vi "Word - Append Table Tests.vi"(8 "error in (no error)":errorcluster) -> (0 "error out":errorcluster)   [LabVIEW 2017]
uses:
  src/LabVIEW NPOI/MS-Word/MS-Word.lvclass
  C:/Users/Neo/Desktop/Dev_Tools_BR/LabVIEW_NPOI/src/LabVIEW NPOI/Document/Document.lvclass
  src/LabVIEW NPOI/Document/Append Table (string).vi
  src/LabVIEW NPOI/Document/Append Table (double).vi
  <vilib>/addons/_JKI Toolkits/Caraya/classes/Assert/Assert Not Error.vi
  src/LabVIEW NPOI/Document/Document.lvclass
  <vilib>/addons/_JKI Toolkits/Caraya/classes/Test/Test.lvclass
  <vilib>/addons/_JKI Toolkits/Caraya/classes/Assert/Assert.lvclass
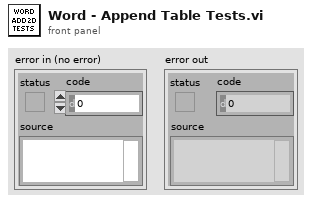
[diagram p1: front panel]
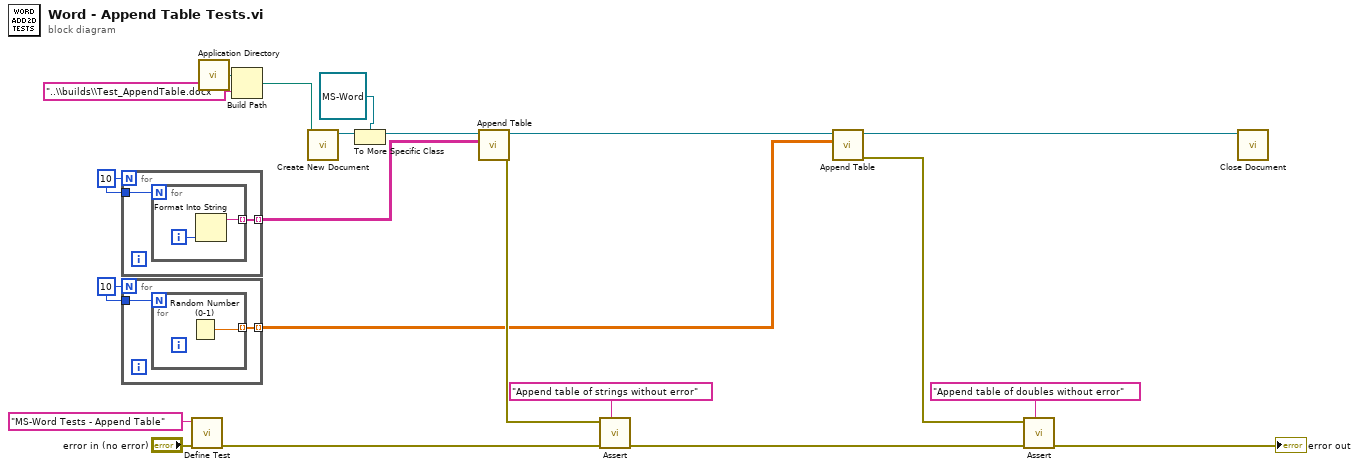
[diagram p0: block diagram]
diagram:
  w8 = 10
  w12 = 10
  n1 = for {
    N: w12 -> [_]
    tunnel: [w23] -> w10 mode=indexing
    tunnel: w12 -> [w22]
    n2 = for {
      N: w22 -> [_]
      tunnel: [w24] -> w23 mode=indexing
      i -> [w25]
      n3 = Format Into String(w25) -> (resulting string=w24:string)  [unwired: 3 in, 1 out]
    }
  }
  n4 = for {
    N: w8 -> [_]
    tunnel: [w27] -> w7 mode=indexing
    tunnel: w8 -> [w26]
    n5 = for {
      N: w26 -> [_]
      tunnel: [w28] -> w27 mode=indexing
      n6 = Random Number (0-1)() -> (number: 0 to 1=w28:dbl)
    }
  }
  n7 = call <vilib>:"Define Test.vi"("error in (no error)"="error in (no error)", "Label (VI Title)"="MS-Word Tests - Append Table") -> ("error out"=w21:errorcluster)  [unwired: 9 in]
  n8 = call <vilib>:"Application Directory.vi"() -> ("Application Directory"=w16:path)
  n9 = Build Path(base path=w16, name or relative path="..\\builds\\Test_AppendTable.docx" ("string")) -> (appended path=w3:path)
  n10 = call "Create New Document.vi"("File Path"=w3) -> ("Document out"=w14:refnum<class "Document.lvclass">)  [unwired: 9 in, 1 out]
  n11 = To More Specific Class(target class=refnum<class "MS-Word.lvclass"> refnum ("LabVIEW NPOI.lvlib:MS-Word.lvclass"), reference=w14) -> (specific class reference=w2:refnum<class "MS-Word.lvclass">)  [unwired: 1 in, 1 out]
  n12 = call-poly "Append Table.vi"("Table"=w10, "Document in"=w2) -> ("error out"=w11:errorcluster, "Document out"=w13:refnum<class "MS-Word.lvclass">)  [unwired: 8 in]
  n13 = call-poly <vilib>:"Assert.vi"("Label"="Append table of strings without error", "error in (no error)"=w21, "Not Error?"=w11) -> ("error out"=w19:errorcluster)  [unwired: 8 in]
  n14 = call-poly "Append Table.vi"("Table"=w7, "Document in"=w13) -> ("error out"=w4:errorcluster, "Document out"=w9:refnum<class "MS-Word.lvclass">)  [unwired: 8 in]
  n15 = call-poly <vilib>:"Assert.vi"("Label"="Append table of doubles without error", "error in (no error)"=w19, "Not Error?"=w4) -> ("error out"=→"error out":errorcluster)  [unwired: 8 in]
  n16 = call "Close Document.vi"("Document in"=w9) -> ()  [unwired: 10 in, 1 out]
